vi "STD获取用户校准参数.vi"(7 "探头":T1(ring), 8 "error in (no error)":errorcluster caption="错误输入（无错误）", 11 "MB session in":refnum<class "MB_Master.lvclass">) -> (0 "error out":errorcluster caption="错误输出", 2 "输出值":cluster{"K":sgl, "B":sgl}, 3 "MB session out":refnum<class "MB_Master.lvclass">)   [LabVIEW 2016, in "斯坦道多参数.lvlib"]
uses:
  <vilib>/Plasmionique/MB Master/MB_Master/MB_Master.lvclass
  <vilib>/Plasmionique/MB Master/MB Master.lvlib
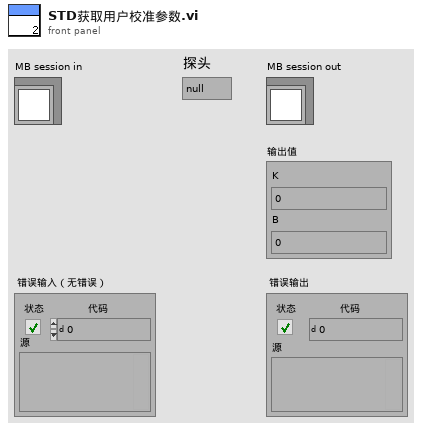
[diagram p1: front panel]
types:
  T1 = enum16{"null", "pH", "DO", "浊度", "电导率", "叶绿素a", "DO2", "藻密度"}
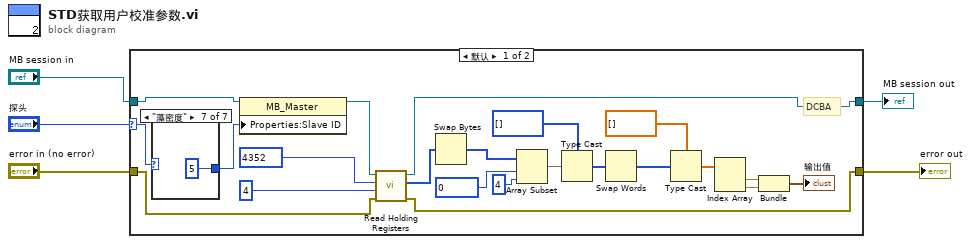
[diagram p0: block diagram]
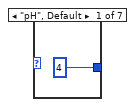
[diagram p2: hidden frame]
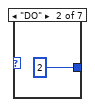
[diagram p3: hidden frame]
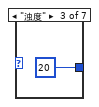
[diagram p4: hidden frame]
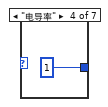
[diagram p5: hidden frame]
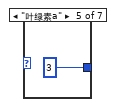
[diagram p6: hidden frame]
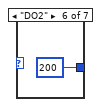
[diagram p7: hidden frame]
diagram:
  n1 = case shown="默认" "探头" {
    selector: "探头" -> [w6 _]
    tunnel: "error in (no error)" -> [w16 w35]
    tunnel: [w14 w35] -> w4
    tunnel: "MB session in" -> [w9 w36]
    tunnel: [w8 w36] -> w2
    frame Default {
      # "DCBA"
      n2 = case shown="\"藻密度\"" w6 {
        tunnel: [u16 4 ("y") u16 2 ("y") u16 20 ("y") u16 1 ("y") u16 3 ("y") u16 200 ("y") u16 5 ("y")] -> w7
        frame "pH", Default {
        }
        frame "DO" {
        }
        frame "浊度" {
        }
        frame "电导率" {
        }
        frame "叶绿素a" {
        }
        frame "DO2" {
        }
        frame "藻密度" {
        }
      }
      n3 = property class="MB_Master"(reference=w9, "Properties:Slave ID"=w7) -> (reference out=w15:refnum<class "MB_Master.lvclass">)  [unwired: 1 in, 1 out]
      n4 = call <vilib>:"Read Holding Registers.vi"("error in (no error)"=w16, "quantity"=u16 4, "starting address"=u16 4352, "MB session in"=w15) -> ("error out"=w14:errorcluster, "Registers"=w13:u16[], "MB session out"=w8:refnum<class "MB_Master.lvclass">)  [unwired: 5 in]
      n5 = Swap Bytes(anything=w13) -> (byte swapped=w12:u16[])
      n6 = Array Subset(array=w12, index=u16 0 ("starting address"), length=4 ("长度")) -> (w11:u16[])
      n7 = Type Cast(type=u32[] [] ("数组 2"), x=w11) -> (*(type *) &x=w22:u32[])
      n8 = Swap Words(1:w22) -> (0:w24:u32[])
      n9 = Type Cast(type=sgl[] [] ("数组 2"), x=w24) -> (*(type *) &x=w20:sgl[])
      n10 = Index Array(array=w20) -> (element #1=w19:sgl, element #2=w18:sgl)  [unwired: 2 in]
      n11 = Bundle("数值"=w19, "数值"=w18) -> (→"输出值":cluster{"数值":sgl, "数值":sgl})  [unwired: 1 in]
    }
    frame "null" {
    }
  }
  "error out" <- w4
  "MB session out" <- w2
